vi "UpdateMenus (SubVI).vi"(7 "UpdateMenuCommand":T1, 8 "Error In":errorcluster) -> (0 "Error Out":errorcluster, 2 "Right Menu":T2, 3 "Left Menu":T2)   [LabVIEW 2017]
doc: "This VI outputs Left and Right Menus for the ATM fron panel depending on the UpdateMenuCommand sent."
uses:
  Controls/Menu.ctl
  Controls/UpdateMenuCommand.ctl
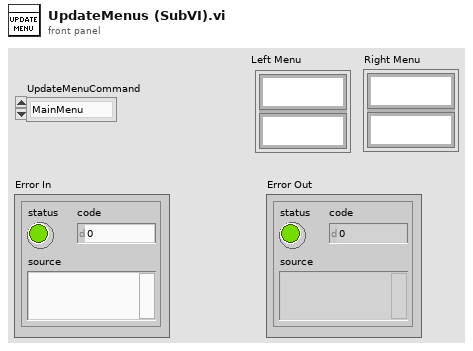
[diagram p1: front panel]
types:
  T1 = typedef "UpdateMenuCommand.ctl" = enum16{"MainMenu", "NoMenu"}
  T2 = typedef "Menu.ctl" = cluster{"Menu 0":string, "Menu 1":string}
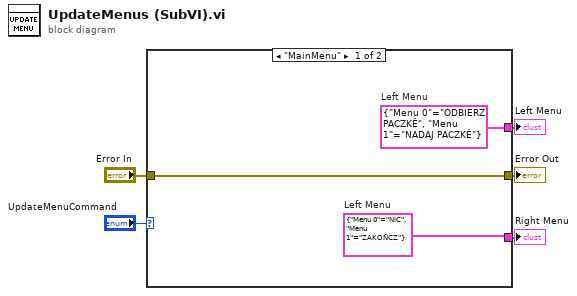
[diagram p0: block diagram]
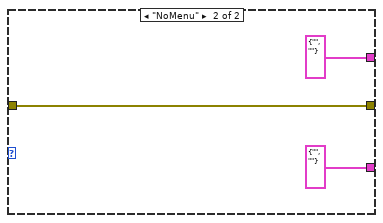
[diagram p2: hidden frame]
diagram:
  n1 = case shown="\"MainMenu\"" "UpdateMenuCommand" {
    tunnel: "Error In" -> [w8 w11]
    tunnel: [w8 w11] -> w4
    tunnel: [w7 T2 {"Menu 0"="", "Menu 1"=""} ("Left Menu")] -> w2
    tunnel: [w6 T2 {"Menu 0"="", "Menu 1"=""} ("Left Menu")] -> w1
    frame "MainMenu" {
      w6 = T2 {"Menu 0"="NIC", "Menu 1"="ZAKOÑCZ"}  # Left Menu
      w7 = T2 {"Menu 0"="ODBIERZ PACZKÊ", "Menu 1"="NADAJ PACZKÊ"}  # Left Menu
    }
    frame "NoMenu" {
    }
  }
  "Error Out" <- w4
  "Left Menu" <- w2
  "Right Menu" <- w1
